vi "Vol-Force_Tuning.vi"() -> ()   [LabVIEW 2016]
uses:
  Classes/DataLogger/Data Logger.lvclass
  <vilib>/Platform/TimedLoop/XDataNode/timing_clust.ctl
  <vilib>/Platform/TimedLoop/XDataNode/nitl_modes.ctl
  <vilib>/Platform/TimedLoop/XDataNode/wakeup.ctl
  <vilib>/DAQmx/read.llb/DAQmx Read (Analog 2D DBL NChan NSamp).vi
  <vilib>/Analysis/baseanly.llb/Mean (DBL).vi
  <vilib>/FPGAPlugInAG/PXI-7842R/niLvFpga_Open_PXI-7842R.vi
  <vilib>/rvi/interface/common/dynamic/niFpgaDynamicAddResources.vi
  <vilib>/FPGAPlugInAG/Dynamic/niLvFpga_Reset_Dynamic.vi
  <vilib>/FPGAPlugInAG/Dynamic/niLvFpga_Run_Dynamic.vi
  <vilib>/Utility/error.llb/Error Cluster From Error Code.vi
  <vilib>/rvi/errors/niLvFpgaAdjustHostInterfaceError.vi
  <vilib>/addons/control/pid/pid.llb/PID Control Input Filter (DBL).vi
  <vilib>/addons/control/pid/pid.llb/PID Advanced (DBL).vi
  <vilib>/addons/control/pid/pid.llb/PID Output Rate Limiter (DBL).vi
  <vilib>/DAQmx/miscellaneous.llb/DAQmx Fill In Error Info.vi
  <vilib>/FPGAPlugInAG/Dynamic/niLvFpga_Abort_Dynamic.vi
  <vilib>/rvi/interface/nirviOpenFPGA/nirviOpenFPGA.xnode
  FPGA Bitfiles/CAlex2_FPGATarget_MotorControl_+dy1qhm6Ymw.lvbitx
  FPGA/MotorControl_PWM+AO.vi
  <vilib>/rvi/interface/nirviMethod/nirviMethod.xnode
  <vilib>/rvi/interface/nirviReadWriteControl/nirviReadWriteControl.xnode
  <vilib>/Platform/TimedLoop/XDataNode/XDataNode.xnode
  <vilib>/Platform/TimedLoop/XDataNode/XDNodeRunTimeDep.lvlib
  <vilib>/rvi/interface/Simulation/niFpgaSimulationCallBeginRW.vi
  <vilib>/addons/control/pid/NI_PID_pid.lvlib
  <vilib>/Analysis/NI_AALBase.lvlib
  NiFpgaLv.dll
panel:
  out "Speed(rpm)":dbl
  in  "Vrpm":i32=9
  out "Current(A)":dbl
  in  "Vfb":i32=8
  out "EncdAngle":sgl[](array[numeric])
  in  "stop":bool
  in  "Load Cell":T1(ring)
  in  "MotorAmt":i32=7
  out "Force (N)":dbl
  in  "ProjectFolder":string="MotorTune"
  in  "File Name":string
  in  "End":dbl
  in  "Begin":dbl
  in  "Start":bool
  in  "Step":dbl
  in  "Duration":dbl
  out "Current":cluster{"output":dbl, "Current(A)":dbl}(graph)
  in  "RateLimiter":dbl=100.0 format="%.2f"
  in  "PID":bool=TRUE
  in  "Manual AO":dbl format="%.2f"
  in  "AO":dbl[](array[numeric])
  in  "Zero":bool
  out "Force":cluster{"setpoint":dbl, "Numeric":dbl}(graph)
  in  "setpoint":dbl format="%.2f"
  in  "reinitialize? (F)":bool
  in  "PID gains":T2={"proportional gain (Kc)"=1.0, "integral time (Ti, min)"=0.01, "derivative time (Td, min)"=0.0} {"derivative time (Td, min)" format="%.5f"; "integral time (Ti, min)" format="%.5f"; "proportional gain (Kc)" format="%.5f"}
  in  "output range":cluster{"output high":dbl, "output low":dbl}={"output high"=5.0, "output low"=-5.0} {"output low" format="%.2f"; "output high" format="%.2f"}
  in  "AO Channel":enum16{"1", "2", "3", "4", "5", "6", "7", "8"}(ring)
  in  "Encoder Channel":enum16{"1", "2", "3", "4", "5", "6", "7", "8"}(ring)
  out "AO Value":dbl[](array[numeric]) format="%.3f"
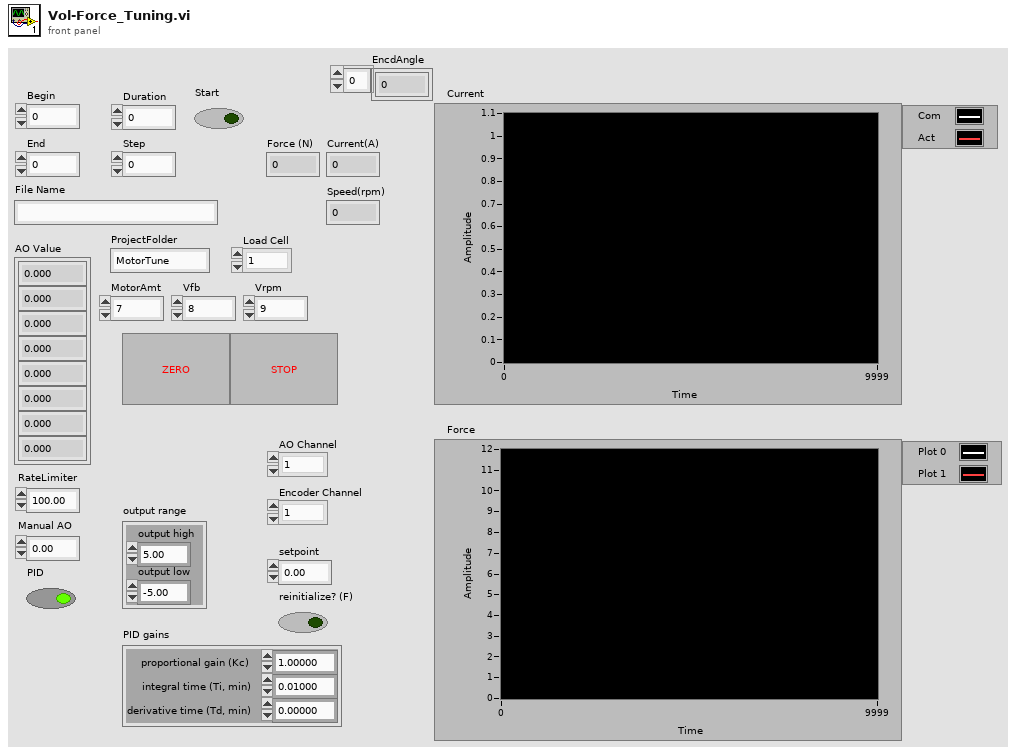
[diagram p1: front panel]
types:
  T1 = enum16{"1", "2", "3", "4", "5", "6", "7", "8", "ai16", "ai17"}
  T2 = cluster{"proportional gain (Kc)":dbl, "integral time (Ti, min)":dbl, "derivative time (Td, min)":dbl}
  T3 = typedef "XDNodeRunTimeDep.lvlib/timing_clust.ctl" = cluster{"Expected End [f-1]":u64, "Actual End [f-1]":u64, "Finished Late? [f-1]":bool, "Expected End [i-1]":u64, "Actual End [i-1]":u64, "Finished Late? [i-1]":bool, "Expected Start [i]":u64, "Actual Start [i]":u64, "Expected Start [f]":u64, "Actual Start [f]":u64, "Source Name":string, "Structure Name":string, "Period":i64, "Deadline":i64, "Offset":i64, "Start":i64, "Priority":i32, "Timeout":i32, "Mode":T4, "Wakeup Reason":T5, "Error":errorcluster, "Source Type":string, "Secondary Source Type":string, "Global End Time":u64, "Global Start Time":u64, "Frame Duration":u64, "Iteration Duration":u64, "Assigned CPU":i32, "I/O Scan Engine Mode":u32}
  T4 = typedef "XDNodeRunTimeDep.lvlib/nitl_modes.ctl" = enum32{"No Change", "Process missed periods, maintain original phase", "Discard missed periods, maintain original phase", "Process missed periods, ignore original phase", "Discard missed periods, ignore original phase"}
  T5 = typedef "XDNodeRunTimeDep.lvlib/wakeup.ctl" = enum32{"Normal", "Aborted", "Asynchronous wakeup", "Timing source error", "Timed loop error", "Timeout"}
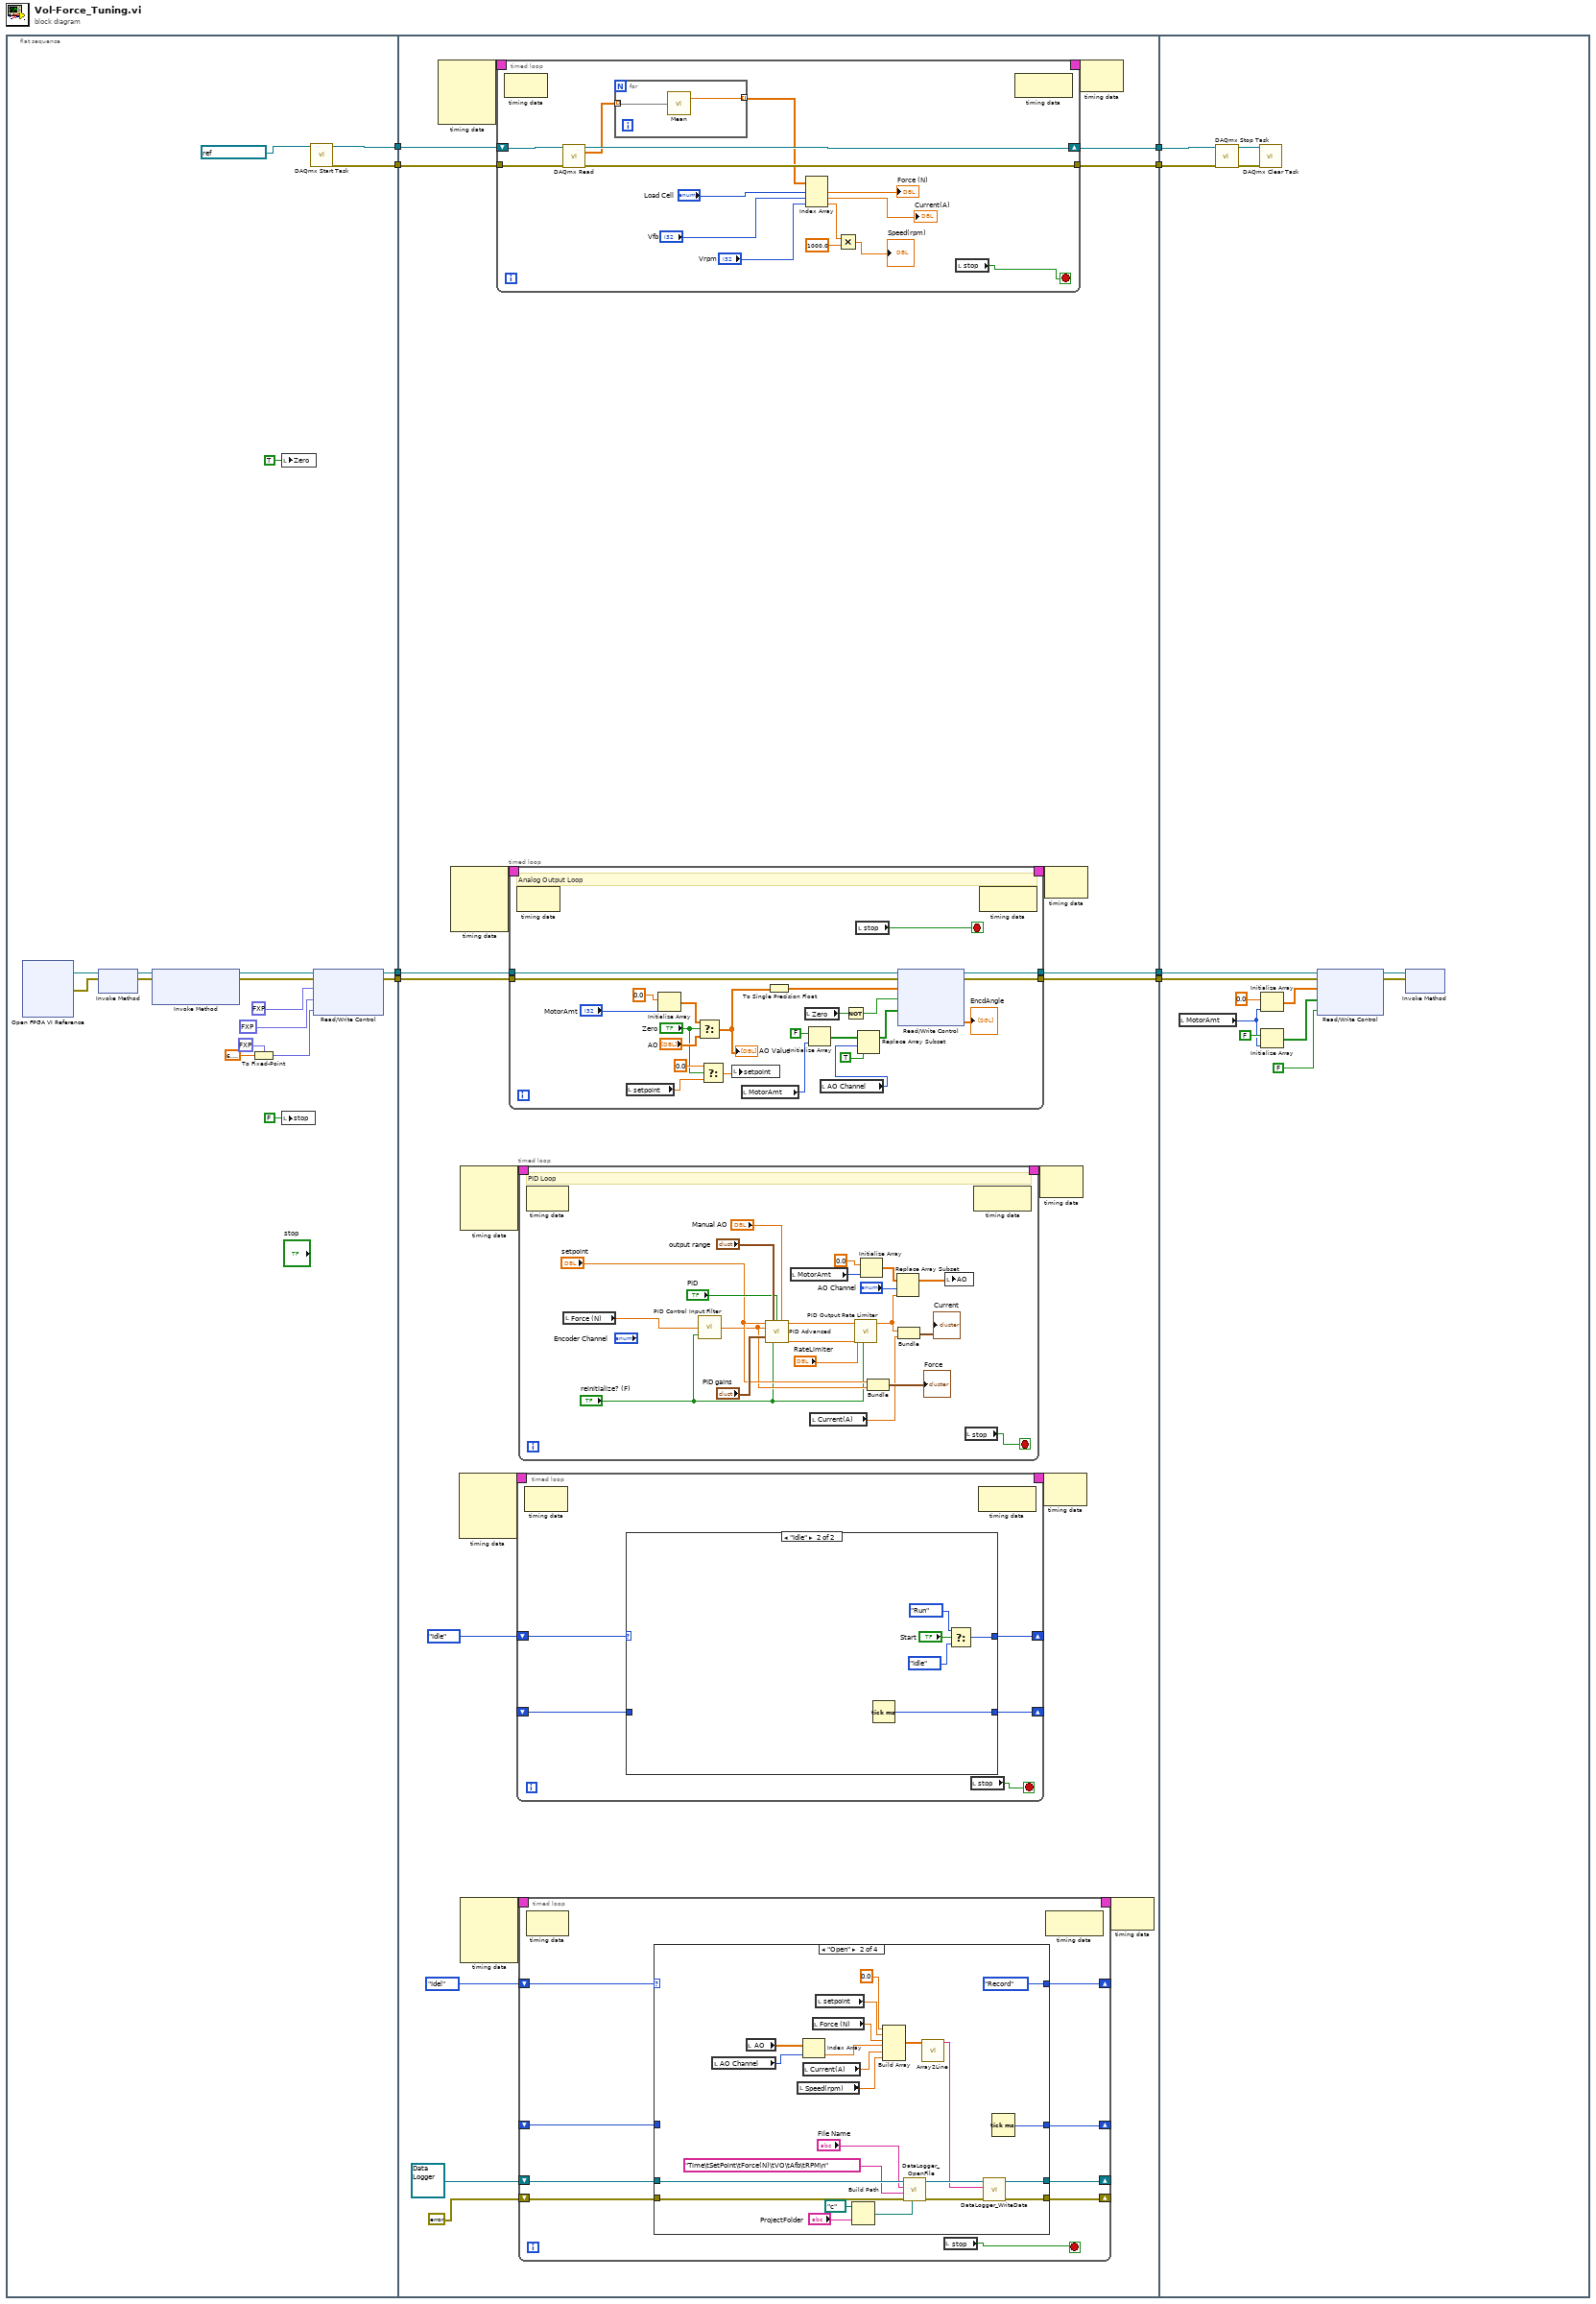
[diagram p0: block diagram]
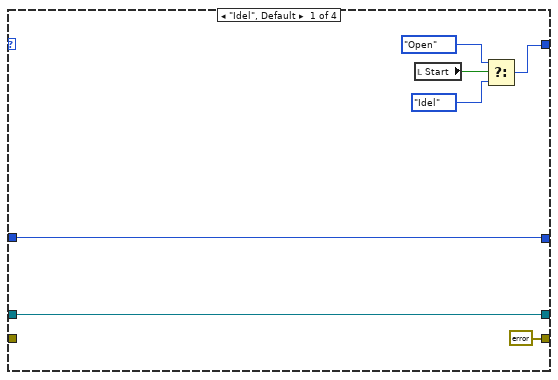
[diagram p2: hidden frame]
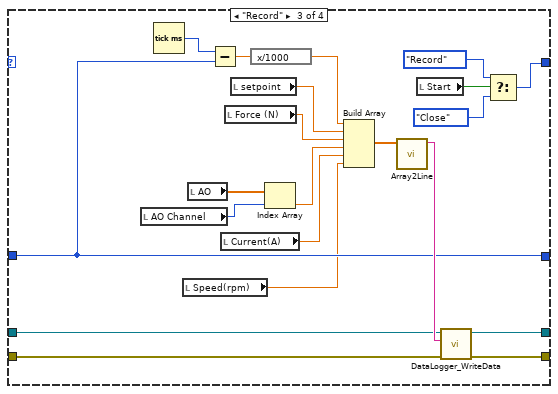
[diagram p3: hidden frame]
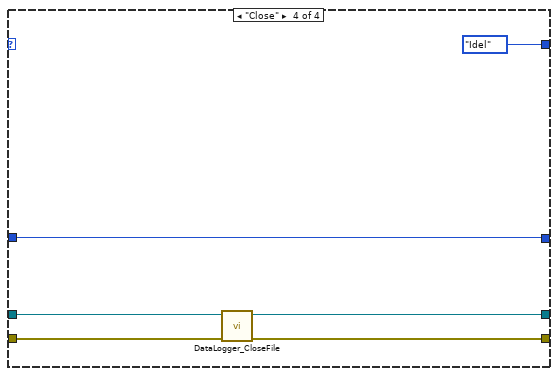
[diagram p4: hidden frame]
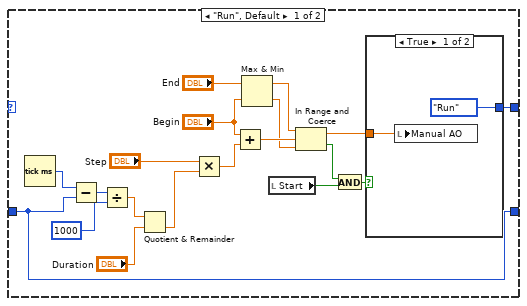
[diagram p5: hidden frame]
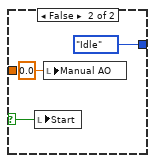
[diagram p6: hidden frame]
diagram:
  n1 = flat-sequence {
    tunnel: [w17] -> w8
    tunnel: [w18] -> w7
    tunnel: [w23] -> w4
    tunnel: [w22] -> w1
    tunnel: w8 -> [w46]
    tunnel: w7 -> [w45]
    tunnel: [w44] -> w6
    tunnel: [w43] -> w5
    tunnel: w4 -> [w30]
    tunnel: [w29] -> w3
    tunnel: [w27] -> w2
    tunnel: w1 -> [w28]
    tunnel: w6 -> [w243]
    tunnel: w5 -> [w244]
    tunnel: w3 -> [w242]
    tunnel: w2 -> [w241]
    frame #0 {
      n2 = xnode "Open FPGA VI Reference"() -> ("FPGA VI Reference Out"=w10:refnum<k20>, "error out"=w9:errorcluster)  [unwired: 2 in]
      n3 = xnode "Invoke Method"("FPGA VI Reference In"=w10, "error in"=w9) -> ("FPGA VI Reference Out"=w26:refnum<k20>, "error out"=w25:errorcluster)
      n4 = xnode "Invoke Method"("FPGA VI Reference In"=w26, "error in"=w25) -> ("FPGA VI Reference Out"=w16:refnum<k20>, "error out"=w19:errorcluster)  [unwired: 1 in]
      n5 = To Fixed-Point(fixed-point type=fxp<+/-,32,10> 0.0 ("2pi"), number=6.283185307179586) -> (fixed-point=w13:fxp<+/-,32,10>)
      n6 = local write "Zero"(TRUE ("Zero")) -> ()
      n7 = local write "stop"(FALSE ("stop")) -> ()
      n8 = call <vilib>:"DAQmx Start Task.vi"("task/channels in"=refnum<k21> "TuningTask" ("Analog Input Channels")) -> ("task out"=w23:refnum<k21>, "error out"=w22:errorcluster)  [unwired: 13 in]
      n9 = xnode "Read/Write Control"("FPGA VI Reference In"=w16, "error in"=w19, "PWM (Hz/A)"=fxp<+/-,32,16> 20.0 ("PWM (Hz/A) 2"), "EncoderCount"=fxp<+,16,16> 500.0 ("EncoderCount 2"), "2pi"=w13) -> ("FPGA VI Reference Out"=w17:refnum<k20>, "error out"=w18:errorcluster)
    }
    frame #1 {
      n10 = node-c288() -> (w32:T3)  [unwired: 4 in]
      n11 = node-c288() -> (w48:T3)  [unwired: 4 in]
      n12 = node-c288() -> (w40:T3)  [unwired: 4 in]
      n13 = node-c288() -> (w42:T3)  [unwired: 4 in]
      n14 = node-c288() -> (w37:T3)  [unwired: 4 in]
      n15 = timed-loop {
        timing: w32 -> [_]
        timing-out: [_] -> w31
        shift-right: [w62] -> w29
        shift-left: w30 -> [w63]
        tunnel: w28 -> [w60]
        tunnel: [w59] -> w27
        stop <- w57 stop-if-true
        n16 = node-c288() -> ()  [unwired: 1 in, 1 out]
        n17 = call-poly <vilib>:"DAQmx Read.vi"("task/channels in"=w63, "error in"=w60) -> ("task out"=w62:refnum<k21>, "data"=w50:dbl[][], "error out"=w59:errorcluster)  [unwired: 11 in]
        n18 = for {
          tunnel: w50 -> [w65] mode=indexing
          tunnel: [w64] -> w49 mode=indexing
          n19 = call-poly <vilib>:"Mean.vi"("X"=w65) -> ("mean"=w64:dbl)  [unwired: 1 out]
        }
        n20 = Index Array(array=w49, index #1="Load Cell", index #2="Vfb", index #3="Vrpm") -> (element #1=→"Force (N)":dbl, element #2=→"Current(A)":dbl, element #3=w53:dbl)
        n21 = Multiply(x=w53, y=1000.0) -> (x*y=→"Speed(rpm)":dbl)
        n22 = local read "stop"() -> (w57:bool)
        n23 = node-c288() -> ()  [unwired: 1 in, 1 out]
      }
      n24 = timed-loop {
        timing: w48 -> [_]
        timing-out: [_] -> w47
        tunnel: w46 -> [w226]
        tunnel: w45 -> [w225]
        tunnel: [w224] -> w43
        tunnel: [w223] -> w44
        stop <- w204 stop-if-true
        # "Analog Output Loop"
        n25 = node-c288() -> ()  [unwired: 1 in, 1 out]
        n26 = local read "setpoint"() -> (w214:dbl)
        n27 = Initialize Array(0.0 ("element"), "MotorAmt") -> (w220:dbl[])
        n28 = Select(t=w220, s="Zero", f="AO") -> (s? t:f=w217:dbl[])
        "AO Value" <- w217
        n29 = Select(t=0.0 ("element"), s="Zero", f=w214) -> (s? t:f=w216:dbl)
        n30 = local write "setpoint"(w216) -> ()
        n31 = local read "MotorAmt"() -> (w209:i32)
        n32 = To Single Precision Float(number=w217) -> (single precision float=w218:sgl[])
        n33 = local read "Zero"() -> (w211:bool)
        n34 = Initialize Array(FALSE, w209) -> (w208:bool[])
        n35 = local read "AO Channel"() -> (w205:enum16{"1", "2", "3", "4", "5", "6", "7", "8"})
        n36 = Not(x=w211) -> (.not. x?=w212:bool)
        n37 = local read "stop"() -> (w204:bool)
        n38 = Replace Array Subset(array=w208, new element=TRUE ("new element/subarray"), index=w205) -> (w207:bool[])
        n39 = xnode "Read/Write Control"("FPGA VI Reference In"=w226, "error in"=w225, "AmpCmd"=w218, "EnableMaster"=w212, "Enable"=w207) -> ("FPGA VI Reference Out"=w224:refnum<k20>, "error out"=w223:errorcluster, "EncdAngle"=→"EncdAngle":sgl[])
        n40 = node-c288() -> ()  [unwired: 1 in, 1 out]
      }
      n41 = timed-loop {
        timing: w40 -> [_]
        timing-out: [_] -> w39
        shift-right: [w141] -> _
        shift-left: enum16{"Run", "Idle"}."Idle" -> [w144]
        shift-right: [w143] -> _
        shift-left: _ -> [w142]
        stop <- w140 stop-if-true
        n42 = node-c288() -> ()  [unwired: 1 in, 1 out]
        n43 = case shown="\"Idle\"" w144 {
          tunnel: [w148 w173] -> w143
          tunnel: w142 -> [w148 _]
          tunnel: [w146 w171] -> w141
          frame "Run", Default {
            n44 = Tick Count (ms)() -> (millisecond timer value=w163:u32)
            n45 = Subtract(x=w163, y=w148) -> (x-y=w162:u32)
            n46 = Divide(x=w162, y=u32 1000) -> (x/y=w159:dbl)
            n47 = Quotient & Remainder(x=w159, y="Duration") -> (floor(x/y)=w157:dbl)  [unwired: 1 out]
            n48 = Multiply(x="Step", y=w157) -> (x*y=w156:dbl)
            n49 = Add(x="Begin", y=w156) -> (x+y=w155:dbl)
            n50 = Max & Min(x="End", y="Begin") -> (max(x,y)=w152:dbl, min(x,y)=w151:dbl)
            n51 = local read "Start"() -> (w150:bool)
            n52 = In Range and Coerce(upper limit=w152, x=w155, lower limit=w151) -> (coerced(x)=w145:dbl, In Range?=w149:bool)
            n53 = And(x=w149, y=w150) -> (x .and. y?=w147:bool)
            n54 = case shown="True" w147 {
              selector: w147 -> [_ w166]
              tunnel: [enum16{"Run", "Idle"}."Run" enum16{"Run", "Idle"}."Idle"] -> w146
              tunnel: w145 -> [w164 _]
              frame True {
                n55 = local write "Manual AO"(w164) -> ()
              }
              frame False {
                n56 = local write "Start"(w166) -> ()
                n57 = local write "Manual AO"(0.0 ("f")) -> ()
              }
            }
          }
          frame "Idle" {
            n58 = Tick Count (ms)() -> (millisecond timer value=w173:u32)
            n59 = Select(t=enum16{"Run", "Idle"}."Run", s="Start", f=enum16{"Run", "Idle"}."Idle") -> (s? t:f=w171:enum16{"Run", "Idle"})
          }
        }
        n60 = local read "stop"() -> (w140:bool)
        n61 = node-c288() -> ()  [unwired: 1 in, 1 out]
      }
      n62 = timed-loop {
        timing: w42 -> [_]
        timing-out: [_] -> w41
        stop <- w179 stop-if-true
        # "PID Loop"
        n63 = node-c288() -> ()  [unwired: 1 in, 1 out]
        n64 = local read "Force (N)"() -> (w181:dbl)
        n65 = call-poly <vilib>:"PID Control Input Filter.vi"("reinitialize? (F)"="reinitialize? (F)", "input"=w181) -> ("output"=w183:dbl)  [unwired: 3 in]
        n66 = call-poly <vilib>:"PID Advanced.vi"("setpoint"="setpoint", "output range"="output range", "auto? (T)"="PID", "manual control"="Manual AO", "process variable"=w183, "PID gains"="PID gains", "reinitialize? (F)"="reinitialize? (F)") -> ("output"=w189:dbl, "dt out (s)"=w188:dbl)  [unwired: 7 in]
        n67 = local read "MotorAmt"() -> (w180:i32)
        n68 = local read "Current(A)"() -> (w178:dbl)
        n69 = call-poly <vilib>:"PID Output Rate Limiter.vi"("reinitialize? (F)"="reinitialize? (F)", "dt (s)"=w188, "output rate (EGU/min)"="RateLimiter", "input (controller output)"=w189) -> ("output"=w184:dbl)  [unwired: 4 in, 1 out]
        n70 = Initialize Array(0.0 ("element"), w180) -> (w196:dbl[])
        n71 = Bundle("setpoint"="setpoint", "output"=w183) -> (→"Force":cluster{"setpoint":dbl, "output":dbl})  [unwired: 1 in]
        n72 = Replace Array Subset(array=w196, new element=w184, index="AO Channel") -> (w197:dbl[])
        n73 = Bundle("output"=w184, "Current(A)"=w178) -> (→"Current":cluster{"output":dbl, "Current(A)":dbl})  [unwired: 1 in]
        n74 = local write "AO"(w197) -> ()
        n75 = local read "stop"() -> (w179:bool)
        n76 = node-c288() -> ()  [unwired: 1 in, 1 out]
      }
      n77 = timed-loop {
        timing: w37 -> [_]
        timing-out: [_] -> w36
        shift-right: [w76] -> _
        shift-left: refnum<class "Data Logger.lvclass"> refnum ("Data Logger out") -> [w77]
        shift-right: [w75] -> _
        shift-left: errorcluster {"status"=FALSE, "code"=0, "source"=""} ("error out") -> [w74]
        shift-right: [w72] -> _
        shift-left: _ -> [w73]
        shift-right: [w71] -> _
        shift-left: enum16{"Close", "Record", "Open", "Idel"}."Idel" -> [w78]
        stop <- w70 stop-if-true
        n78 = node-c288() -> ()  [unwired: 1 in, 1 out]
        n79 = case shown="\"Open\"" w78 {
          tunnel: w77 -> [w85 w108 w121 w135]
          tunnel: [w85 w107 w129 w133] -> w76
          tunnel: [errorcluster {"status"=FALSE, "code"=0, "source"=""} ("error out") w104 w128 w132] -> w75
          tunnel: w74 -> [_ w103 w120 w134]
          tunnel: w73 -> [w80 _ w118 w131]
          tunnel: [w80 w94 w118 w131] -> w72
          tunnel: [w83 enum16{"Close", "Record", "Open", "Idel"}."Record" w114 enum16{"Close", "Record", "Open", "Idel"}."Idel"] -> w71
          frame "Idel", Default {
            n80 = local read "Start"() -> (w84:bool)
            n81 = Select(t=enum16{"Close", "Record", "Open", "Idel"}."Open", s=w84, f=enum16{"Close", "Record", "Open", "Idel"}."Idel") -> (s? t:f=w83:enum16{"Close", "Record", "Open", "Idel"})
          }
          frame "Open" {
            n82 = local read "AO Channel"() -> (w102:enum16{"1", "2", "3", "4", "5", "6", "7", "8"})
            n83 = local read "AO"() -> (w101:dbl[])
            n84 = local read "Speed(rpm)"() -> (w86:dbl)
            n85 = Index Array(array=w101, index=w102) -> (element=w99:dbl)
            n86 = local read "Current(A)"() -> (w87:dbl)
            n87 = local read "Force (N)"() -> (w91:dbl)
            n88 = local read "setpoint"() -> (w100:dbl)
            n89 = Build Path(base path=path "c:/", name or relative path="ProjectFolder") -> (appended path=w90:path)
            n90 = Build Array(0.0 ("element"), w100, w91, w99, w87, w86) -> (w98:dbl[])
            n91 = call "DataLogger_OpenFile.vi"("base path (C:\\CAlex\\)"=w90, "error in (no error)"=w103, "Header"="Time\tSetPoint\tForce(N)\tVO\tAfb\tRPM\n", "File Name"="File Name", "Data Logger in"=w108) -> ("error out"=w105:errorcluster, "Data Logger out"=w106:refnum<class "Data Logger.lvclass">)  [unwired: 5 in]
            n92 = call "Array2Line.vi"("Data"=w98) -> ("String"=w97:string)  [unwired: 10 in]
            n93 = call "DataLogger_WriteData.vi"("error in (no error)"=w105, "New line"=w97, "Data Logger in"=w106) -> ("error out"=w104:errorcluster, "Data Logger out"=w107:refnum<class "Data Logger.lvclass">)  [unwired: 7 in]
            n94 = Tick Count (ms)() -> (millisecond timer value=w94:u32)
          }
          frame "Record" {
            n95 = local read "AO Channel"() -> (w127:enum16{"1", "2", "3", "4", "5", "6", "7", "8"})
            n96 = Tick Count (ms)() -> (millisecond timer value=w119:u32)
            n97 = local read "Speed(rpm)"() -> (w109:dbl)
            n98 = local read "AO"() -> (w126:dbl[])
            n99 = Subtract(x=w119, y=w118) -> (x-y=w113:dbl)
            n100 = local read "Current(A)"() -> (w110:dbl)
            n101 = local read "Force (N)"() -> (w111:dbl)
            n102 = local read "setpoint"() -> (w125:dbl)
            n103 = expression code="x/1000"(w113) -> (w112:dbl)
            n104 = Index Array(array=w126, index=w127) -> (element=w124:dbl)
            n105 = Build Array(w112, w125, w111, w124, w110, w109) -> (w123:dbl[])
            n106 = call "Array2Line.vi"("Data"=w123) -> ("String"=w122:string)  [unwired: 10 in]
            n107 = local read "Start"() -> (w117:bool)
            n108 = call "DataLogger_WriteData.vi"("error in (no error)"=w120, "New line"=w122, "Data Logger in"=w121) -> ("error out"=w128:errorcluster, "Data Logger out"=w129:refnum<class "Data Logger.lvclass">)  [unwired: 7 in]
            n109 = Select(t=enum16{"Close", "Record", "Open", "Idel"}."Record", s=w117, f=enum16{"Close", "Record", "Open", "Idel"}."Close") -> (s? t:f=w114:enum16{"Close", "Record", "Open", "Idel"})
          }
          frame "Close" {
            n110 = call "DataLogger_CloseFile.vi"("error in (no error)"=w134, "Data Logger in"=w135) -> ("error out"=w132:errorcluster, "Data Logger out"=w133:refnum<class "Data Logger.lvclass">)  [unwired: 8 in]
          }
        }
        n111 = local read "stop"() -> (w70:bool)
        n112 = node-c288() -> ()  [unwired: 1 in, 1 out]
      }
      n113 = node-c288(w41) -> ()  [unwired: 1 out]
      n114 = node-c288(w39) -> ()  [unwired: 1 out]
      n115 = node-c288(w47) -> ()  [unwired: 1 out]
      n116 = node-c288(w31) -> ()  [unwired: 1 out]
      n117 = node-c288(w36) -> ()  [unwired: 1 out]
    }
    frame #2 {
      n118 = local read "MotorAmt"() -> (w234:i32)
      n119 = call <vilib>:"DAQmx Stop Task.vi"("task/channels in"=w242, "error in"=w241) -> ("task out"=w232:refnum<k21>, "error out"=w231:errorcluster)  [unwired: 12 in]
      n120 = call <vilib>:"DAQmx Clear Task.vi"("task in"=w232, "error in"=w231) -> ()  [unwired: 13 in, 1 out]
      n121 = Initialize Array(0.0 ("element"), w234) -> (w239:dbl[])
      n122 = Initialize Array(FALSE, w234) -> (w236:bool[])
      n123 = xnode "Read/Write Control"("FPGA VI Reference In"=w244, "error in"=w243, "AmpCmd"=w239, "Enable"=w236, "EnableMaster"=FALSE) -> ("FPGA VI Reference Out"=w238:refnum<k20>, "error out"=w237:errorcluster)
      n124 = xnode "Invoke Method"("FPGA VI Reference In"=w238, "error in"=w237) -> ()  [unwired: 2 out]
    }
  }
